vi "Equal.vi"(9 "Semver 2":refnum<class "Semver.lvclass">, 10 "Semver 1":refnum<class "Semver.lvclass">) -> (2 "Version 1 = Version 2":bool)   [LabVIEW 2017, in "Semver.lvlib" / "Semver.lvclass"]
uses:
  Semver.lvclass
  Semver.lvclass/Semver.ctl
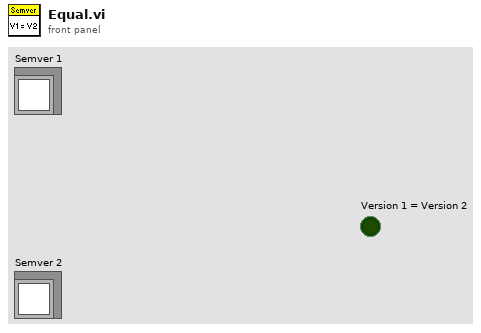
[diagram p1: front panel]
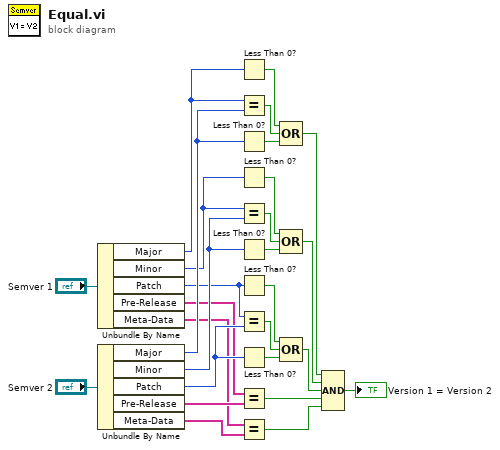
[diagram p0: block diagram]
diagram:
  n1 = Unbundle By Name("Semver 1") -> ("Major"=w25:i32, "Minor"=w16:i32, "Patch"=w11:i32, "Pre-Release"=w7:string[], "Meta-Data"=w5:string[])
  n2 = Unbundle By Name("Semver 2") -> ("Major"=w24:i32, "Minor"=w15:i32, "Patch"=w10:i32, "Pre-Release"=w6:string[], "Meta-Data"=w4:string[])
  n3 = Less Than 0?(x=w25) -> (x < 0?=w23:bool)
  n4 = Equal?(x=w25, y=w24) -> (x = y?=w22:bool)
  n5 = Less Than 0?(x=w24) -> (x < 0?=w21:bool)
  n6 = Less Than 0?(x=w16) -> (x < 0?=w17:bool)
  n7 = Equal?(x=w16, y=w15) -> (x = y?=w18:bool)
  n8 = Less Than 0?(x=w15) -> (x < 0?=w19:bool)
  n9 = Less Than 0?(x=w11) -> (x < 0?=w12:bool)
  n10 = Equal?(x=w11, y=w10) -> (x = y?=w13:bool)
  n11 = Less Than 0?(x=w10) -> (x < 0?=w14:bool)
  n12 = Equal?(x=w7, y=w6) -> (x = y?=w3:bool)
  n13 = Equal?(x=w5, y=w4) -> (x = y?=w2:bool)
  n14 = Compound Arithmetic op=OR(w23, w22, w21) -> (w20:bool)
  n15 = Compound Arithmetic op=OR(w17, w18, w19) -> (w9:bool)
  n16 = Compound Arithmetic op=OR(w12, w13, w14) -> (w8:bool)
  n17 = Compound Arithmetic op=AND(w20, w9, w8, w3, w2) -> (→"Version 1 = Version 2":bool)
